vi "AcquireData.vi"(9 "Velocity":dbl, 10 "Target position":dbl, 11 "Start position":dbl) -> (0 "error out":errorcluster, 2 "data":waveform(dbl), 3 "task out":refnum<k21>)   [LabVIEW 2013]
uses:
  <vilib>/DAQmx/read.llb/DAQmx Read (Analog Wfm 1Chan NSamp).vi
  Global.vi
  <vilib>/DAQmx/miscellaneous.llb/DAQmx Fill In Error Info.vi
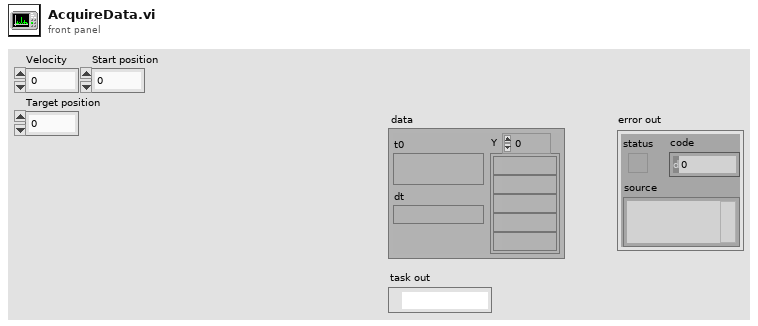
[diagram p1: front panel]
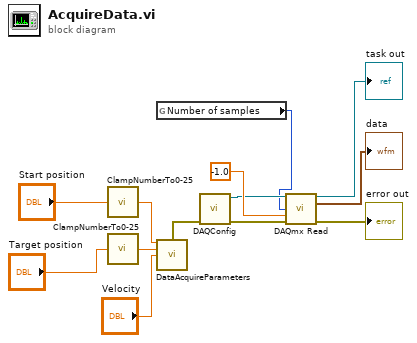
[diagram p0: block diagram]
diagram:
  n1 = call "ClampNumberTo0-25.vi"("Number"="Start position") -> ("Clamped number"=w5:dbl)
  n2 = call "ClampNumberTo0-25.vi"("Number"="Target position") -> ("Clamped number"=w3:dbl)
  n3 = global read "Global.vi" "Number of samples"() -> (w1:i32)
  n4 = call "DataAcquireParameters.vi"("Start position"=w5, "Target position"=w3, "Velocity"="Velocity") -> ("error constant"=w2:errorcluster)  [unwired: 5 in, 7 out]
  n5 = call "DAQConfig.vi"("error in"=w2) -> ("error out"=w9:errorcluster, "task out"=w8:refnum<k21>)  [unwired: 9 in]
  n6 = call-poly <vilib>:"DAQmx Read.vi"("task/channels in"=w8, "number of samples per channel"=w1, "timeout"=-1.0, "error in"=w9) -> ("task out"=→"task out":refnum<k21>, "data"=→"data":waveform(dbl), "error out"=→"error out":errorcluster)  [unwired: 9 in]
